vi "get handler dataset.vi"(8 "error in":errorcluster, 11 "Basic HTTP server in":refnum<class "Basic HTTPS server.lvclass">) -> (0 "error out":errorcluster, 2 "basic HTTP handler dataset":refnum<class "HTTPS handler dataset.lvclass">)   [LabVIEW 2016, in "Basic HTTPS server.lvclass"]
uses:
  Basic HTTPS server.lvclass
  HTTP handler dataset/HTTPS handler dataset.lvclass
  http server info.ctl
  Basic HTTPS server.lvclass/Basic HTTPS server.ctl
  lvlibtls/server/lvlibretls server listener.lvclass
  HTTP handler dataset/HTTPS handler dataset.lvclass/HTTPS handler dataset.ctl
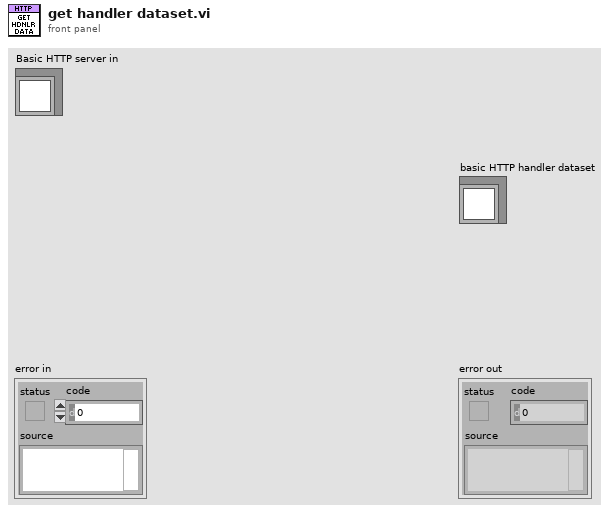
[diagram p1: front panel]
types:
  T1 = typedef "Basic HTTPS server.lvclass/http server info.ctl" = cluster{"port":u16}
  T2 = typedef "Basic HTTPS server.lvclass/http server properties.ctl" = cluster{"max url size":i32, "max header":i32, "timeout ms":i32, "max data size":i32}
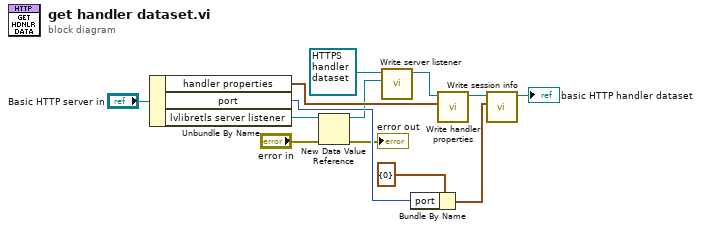
[diagram p0: block diagram]
diagram:
  n1 = Unbundle By Name("Basic HTTP server in") -> ("handler properties"=w12:T2, "port"=w7:u16, "lvlibretls server listener"=w4:refnum<class "lvlibretls server listener.lvclass">)
  n2 = New Data Value Reference(data value=w4, error in="error in") -> (data value reference=w1:refnum<data-value>, error out=→"error out":errorcluster)
  n3 = call "Write server listener.vi"("server listener"=w1, "basic HTTP handler dataset in"=refnum<class "HTTPS handler dataset.lvclass"> refnum) -> ("basic HTTP handler dataset out"=w2:refnum<class "HTTPS handler dataset.lvclass">)  [unwired: 9 in]
  n4 = Bundle By Name(cluster=T1 {"port"=0} ("server information"), "port"=w7) -> (w8:T1)
  n5 = call "Write handler properties.vi"("server properties"=w12, "basic HTTP handler dataset in"=w2) -> ("basic HTTP handler dataset out"=w11:refnum<class "HTTPS handler dataset.lvclass">)  [unwired: 9 in]
  n6 = call "Write session info.vi"("server information"=w8, "basic HTTP handler dataset in"=w11) -> ("basic HTTP handler dataset out"=→"basic HTTP handler dataset":refnum<class "HTTPS handler dataset.lvclass">)  [unwired: 9 in]
